vi "Read Process ID.vi"(0 "Process In":refnum<class "Process.lvclass">, 11 "Error In":errorcluster) -> (4 "Process Out":refnum<class "Process.lvclass">, 6 "Process ID":u32, 15 "Error Out":errorcluster)   [LabVIEW 2023, in "Process.lvclass"]
uses:
  Process.lvclass
  Process.lvclass/Process.ctl
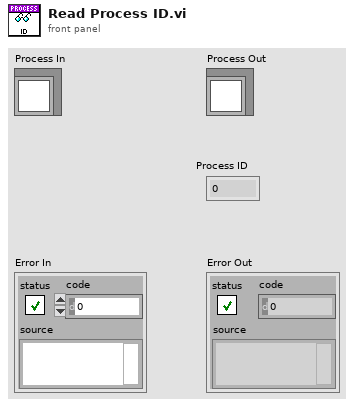
[diagram p1: front panel]
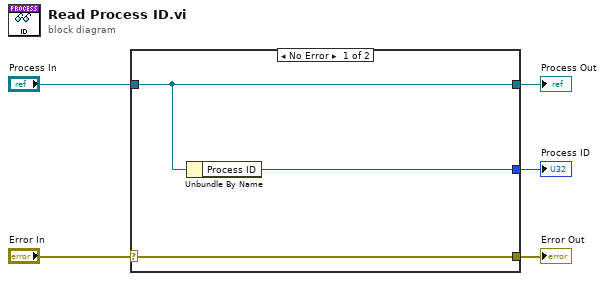
[diagram p0: block diagram]
diagram:
  n1 = case shown="No Error" "Error In" {
    selector: "Error In" -> [w8 w9]
    tunnel: [w8 w9] -> w4
    tunnel: [w7 w10] -> w2
    tunnel: "Process In" -> [w7 w10]
    tunnel: [w6 _] -> w1
    frame No Error {
      n2 = Unbundle By Name(w7) -> ("Process ID"=w6:u32)
    }
    frame Error {
    }
  }
  "Error Out" <- w4
  "Process Out" <- w2
  "Process ID" <- w1
